vi "transmitRFID v5 cw_query_rn16.vi"() -> ()   [LabVIEW 2015]
uses:
  Global_bits.vi
  <instrlib>/niUSRP/niUSRP Write Tx Data (CDB).vi
panel:
  out "bits":i16[](graph)
  out "RN16 array":i32[](array[numeric])
  in  "query":bool
  out "RFID Pushed":bool
  out "error out":errorcluster
  in  "Parameters Query":T1 {"Session" items=["S0", "S1", "S2", "S3"]; "Sel" items=["All", "All2", "~SL", "SL"]; "M" items=["M=1", "M=2", "M=4", "M=8"]}
  out "Waveform Magnitude":dbl[](graph)
  out "Loop":i32
  in  "Symbol Rate [Hz]":dbl=500000.0 format="%#_13p"
  in  "Parameters Select":T2={"Target"=7, "Action"=0, "MemBank"=1, "truncate"=FALSE} {"MemBank" items=["00 RFU", "01 EPC", "10 TID", "11 User"]; "Action" items=["000", "001", "010", "011", "100", "101", "110", "111"]; "Target" items=["000 Inventoried (S0)", "001 Inventoried (S1)", "010 Inventoried (S2)", "011 Inventoried (S3)", "100 SL", "101 RFU", "110 RFU", "111 RFU"]}
  in  "Parameters Symbols":T3={"Tari"=8e-06, "PW"=0.5, "factor for \"1\" symbol"=0.5, "RTcal"=2.5, "TRcal"=3.0, "Delimiter"=1.4e-05} {"TRcal" min=1.1 max=3.0 step=0.1; "RTcal" min=2.5 max=3.0 step=0.1; "factor for \"1\" symbol" min=0.5 max=1.0 step=0.1; "PW" min=0.265 max=0.525 step=0.001; "Tari" format="%#_3p"}
  out "coerced IQ rate":dbl=100000.0 format="%#_6p"
  out "carrier frequency":dbl=100000.0 format="%#_6p"
  out "coerced gain":dbl format="%#_6f"
  in  "stop":bool
  in  "IQ rate":dbl=2000000.0 format="%#_6p"
  in  "carrier frequency":dbl=920000000.0 format="%#_6p"
  in  "gain":dbl format="%#_6f"
  in  "tx device names":refnum<k15>="192.168.20.13"
  # "Transmit RFID"
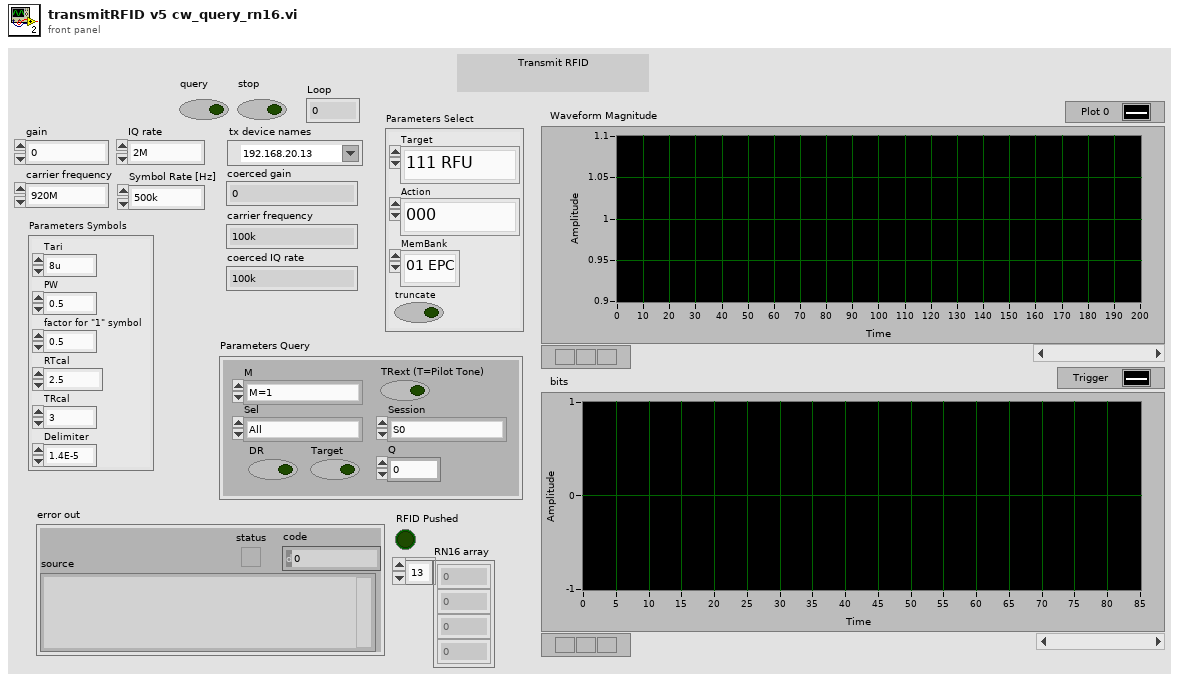
[diagram p1: front panel]
types:
  T1 = cluster{"DR":bool, "M":u16, "TRext (T=Pilot Tone)":bool, "Sel":u16, "Session":u16, "Q":u8, "Target":bool}
  T2 = cluster{"Target":u16, "Action":u16, "MemBank":u16, "truncate":bool}
  T3 = cluster{"Tari":dbl, "PW":dbl, "factor for \"1\" symbol":dbl, "RTcal":dbl, "TRcal":dbl, "Delimiter":dbl}
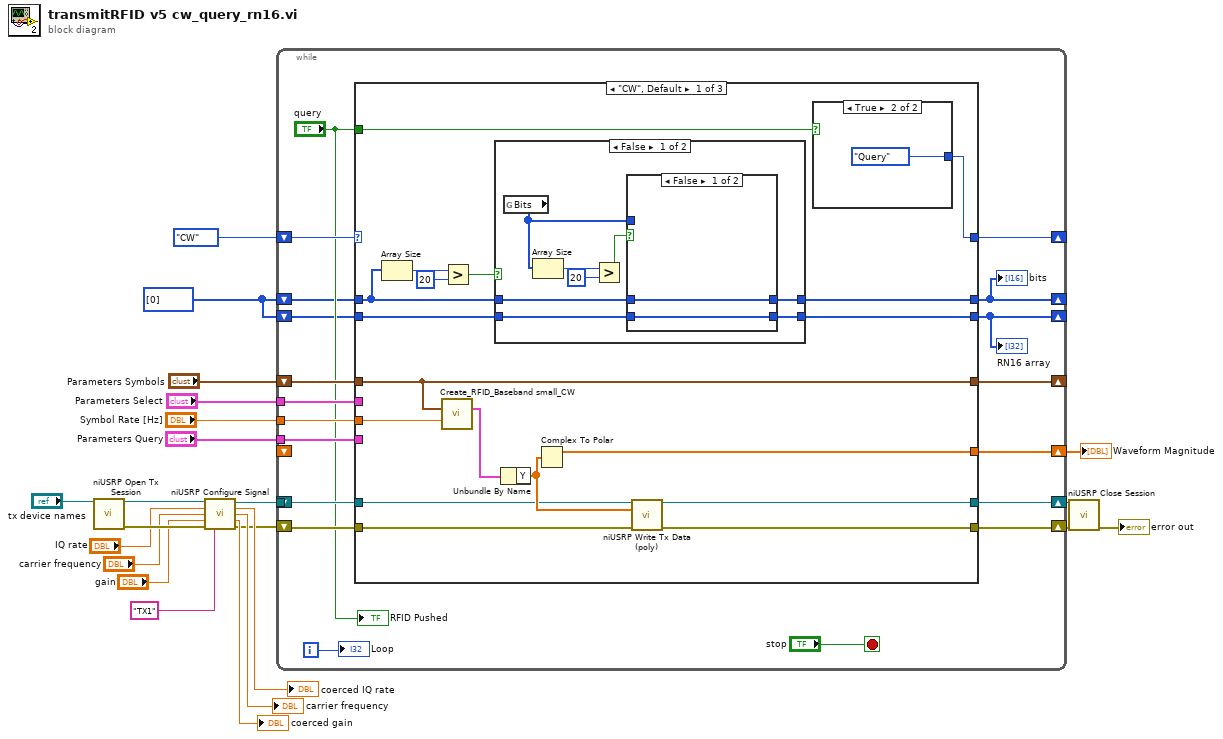
[diagram p0: block diagram]
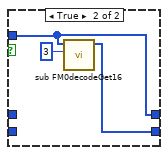
[diagram p2: hidden frame]
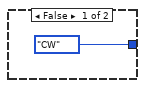
[diagram p4: hidden frame]
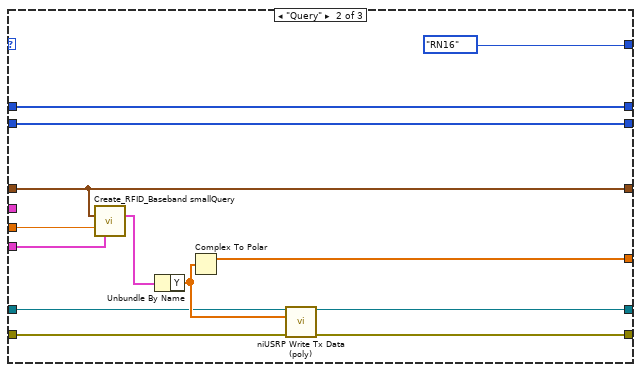
[diagram p5: hidden frame]
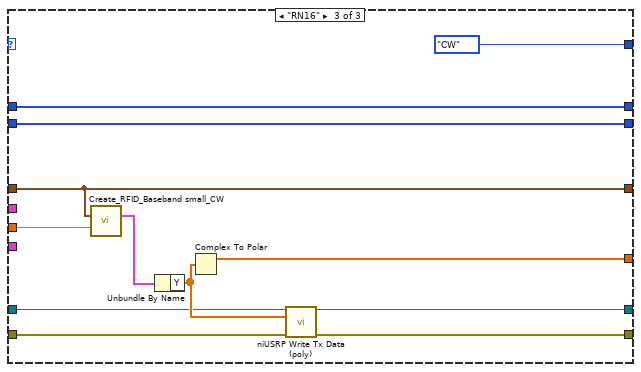
[diagram p6: hidden frame]
diagram:
  w1 = i16[] [0]
  n1 = call <instrlib>:"niUSRP Open Tx Session.vi"("device names"="tx device names") -> ("session handle out"=w2:refnum<k15>, "error out"=w22:errorcluster)  [unwired: 13 in]
  n2 = call <instrlib>:"niUSRP Configure Signal.vi"("session handle"=w2, "IQ rate"="IQ rate", "carrier frequency"="carrier frequency", "gain"="gain", "error in (no error)"=w22, "active antenna"="TX1") -> ("session handle out"=w9:refnum<k15>, "coerced IQ rate"=→"coerced IQ rate":dbl, "coerced carrier frequency"=→"carrier frequency":dbl, "coerced gain"=→"coerced gain":dbl, "error out"=w8:errorcluster)  [unwired: 5 in]
  n3 = while {
    tunnel: "Parameters Select" -> [w34]
    tunnel: "Parameters Query" -> [w32]
    tunnel: w9 -> [w39]
    shift-right: [w37] -> w7
    shift-left: w8 -> [w38]
    shift-right: [w36] -> w5
    shift-left: _ -> [_]
    shift-right: [w28] -> _
    shift-left: enum16{"CW", "Query", "RN16"}."CW" -> [w40]
    shift-right: [w31] -> _
    shift-left: "Parameters Symbols" -> [w35]
    shift-right: [w29] -> w3
    shift-left: _ -> [_]
    tunnel: "Symbol Rate [Hz]" -> [w33]
    shift-right: [w25] -> _
    shift-left: w1 -> [w26]
    shift-right: [w24] -> _
    shift-left: w1 -> [w23]
    i -> [w41]
    stop <- "stop" stop-if-true
    n4 = case shown="\"CW\", Default" w40 {
      tunnel: w39 -> [w58 w88 w100]
      tunnel: w38 -> [w57 w87 w99]
      tunnel: [w56 w86 w98] -> w37
      tunnel: [w55 w85 w97] -> w36
      tunnel: w35 -> [w53 w80 w93]
      tunnel: w34 -> [_ _ _]
      tunnel: w33 -> [w52 w81 w94]
      tunnel: w32 -> [_ w82 _]
      tunnel: [w53 w80 w93] -> w31
      tunnel: [w54 w84 w96] -> w29
      tunnel: [w50 enum16{"CW", "Query", "RN16"}."RN16" enum16{"CW", "Query", "RN16"}."CW"] -> w28
      tunnel: "query" -> [w49 _ _]
      tunnel: w26 -> [w44 w78 w91]
      tunnel: [w45 w78 w91] -> w25
      tunnel: [w43 w77 w90] -> w24
      tunnel: w23 -> [w42 w77 w90]
      frame "CW", Default {
        n5 = Array Size(array=w44) -> (size(s)=w48:i32)
        n6 = call "Create_RFID_Baseband small_CW.vi"("Parameters Symbols"=w53, "Symbol Rate [Hz]"=w52) -> ("complex waveform"=w51:cluster{"t0":dbl, "dt":dbl, "Y":cdb[]})  [unwired: 12 in, 1 out]
        n7 = Greater?(x=w48, y=20) -> (0:w46:bool)
        n8 = case shown="False" w46 {
          tunnel: [w63 w74] -> w45
          tunnel: w44 -> [w64 w74]
          tunnel: [w61 w73] -> w43
          tunnel: w42 -> [w60 w73]
          frame False {
            n9 = global read "Global_bits.vi" "Bits"() -> (w62:i16[])
            n10 = Array Size(array=w62) -> (size(s)=w67:i32)
            n11 = Greater?(x=w67, y=20) -> (0:w65:bool)
            n12 = case shown="False" w65 {
              tunnel: w64 -> [w69 _]
              tunnel: [w69 w71] -> w63
              tunnel: w62 -> [_ w71]
              tunnel: [w68 w70] -> w61
              tunnel: w60 -> [w68 _]
              frame False {
              }
              frame True {
                n13 = call "sub FM0decodeGet16.vi"("threshold"=3, "RN16 waveform"=w71) -> ("RN16 array"=w70:i32[])  [unwired: 9 in]
              }
            }
          }
          frame True {
          }
        }
        n14 = Unbundle By Name(w51) -> ("Y"=w59:cdb[])
        n15 = Complex To Polar(r * e^(i*theta)=w59) -> (r=w54:dbl[])  [unwired: 1 out]
        n16 = call-poly <instrlib>:"niUSRP Write Tx Data (poly).vi"("session handle"=w58, "data"=w59, "error in (no error)"=w57) -> ("session handle out"=w55:refnum<k15>, "error out"=w56:errorcluster)  [unwired: 11 in]
        n17 = case shown="True" w49 {
          tunnel: [enum16{"CW", "Query", "RN16"}."CW" enum16{"CW", "Query", "RN16"}."Query"] -> w50
          frame False {
          }
          frame True {
          }
        }
      }
      frame "Query" {
        n18 = call "Create_RFID_Baseband smallQuery.vi"("Parameters Symbols"=w80, "Symbol Rate [Hz]"=w81, "Parameters Query"=w82) -> ("complex waveform"=w83:cluster{"t0":dbl, "dt":dbl, "Y":cdb[]})  [unwired: 11 in, 1 out]
        n19 = Unbundle By Name(w83) -> ("Y"=w89:cdb[])
        n20 = Complex To Polar(r * e^(i*theta)=w89) -> (r=w84:dbl[])  [unwired: 1 out]
        n21 = call-poly <instrlib>:"niUSRP Write Tx Data (poly).vi"("session handle"=w88, "data"=w89, "error in (no error)"=w87) -> ("session handle out"=w85:refnum<k15>, "error out"=w86:errorcluster)  [unwired: 11 in]
      }
      frame "RN16" {
        n22 = call "Create_RFID_Baseband small_CW.vi"("Parameters Symbols"=w93, "Symbol Rate [Hz]"=w94) -> ("complex waveform"=w95:cluster{"t0":dbl, "dt":dbl, "Y":cdb[]})  [unwired: 12 in, 1 out]
        n23 = Unbundle By Name(w95) -> ("Y"=w101:cdb[])
        n24 = Complex To Polar(r * e^(i*theta)=w101) -> (r=w96:dbl[])  [unwired: 1 out]
        n25 = call-poly <instrlib>:"niUSRP Write Tx Data (poly).vi"("session handle"=w100, "data"=w101, "error in (no error)"=w99) -> ("session handle out"=w97:refnum<k15>, "error out"=w98:errorcluster)  [unwired: 11 in]
      }
    }
    "RN16 array" <- w24
    "bits" <- w25
    "Loop" <- w41
    "RFID Pushed" <- "query"
  }
  "Waveform Magnitude" <- w3
  n26 = call <instrlib>:"niUSRP Close Session.vi"("session handle"=w5, "error in (no error)"=w7) -> ("error out"=→"error out":errorcluster)  [unwired: 13 in]
